vi "Obtain Priority Queue.vi"(8 "error in (no error)":errorcluster, 9 "Create If Not Found? (T)":bool=TRUE) -> (0 "error out":errorcluster, 1 "Created New?":bool, 3 "Priority Queue":T1)   [LabVIEW 2017, in "Communicable State Machine.lvlib"]
doc: "### Obtain Priority Queue.vi\n\n-- <b>Controls</b> --\n- <b>create if not found? (T)</b>:\n- <b>name</b>:\n\n-- <b>Indicators</b> --\n- <b>created new?</b>:\n- <b>Priority Queue</b>:"
uses:
  Communicable State Machine.lvlib
  Priority Queue.ctl
  Typedef/_Cross CSM State Data.ctl
  Typedef/_CSM_MSG_TYPE.ctl
  Typedef/_Cross CSM State Response.ctl
  Typedef/_CSM_Response Source Message.ctl
  def-Data(LowPRI-Q).ctl
panel:
  in  "Name":string
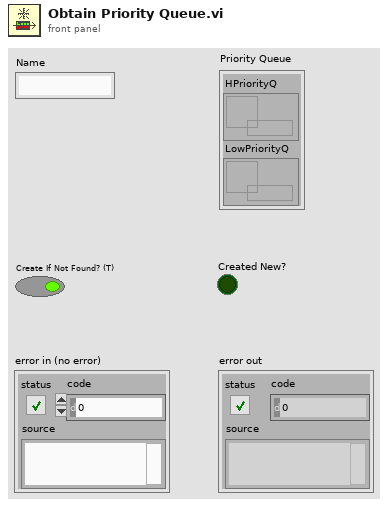
[diagram p1: front panel]
types:
  T1 = typedef "Communicable State Machine.lvlib/Priority Queue.ctl" = cluster{"HPriorityQ":refnum<queue>, "LowPriorityQ":refnum<queue>}
  T2 = typedef "Communicable State Machine.lvlib/def-Data(LowPRI-Q).ctl" = cluster{"Data":T3, "Notify?":bool}
  T3 = typedef "Communicable State Machine.lvlib/_Cross CSM State Data.ctl" = cluster{"Msg Type":T4, "state":string, "args":string, "source":string, "RespQ":refnum<queue>, "Response For Message":T5, "Target":string}
  T4 = typedef "Communicable State Machine.lvlib/_CSM_MSG_TYPE.ctl" = enum16{"Sync Message(-@)", "Async Message(->)", "Async without Response(->|)", "Async Response", "Broadcast(-><all>)", "Broadcast(-><status>)", "Broadcast(-><interrupt>)", "Append to JKISM States", "Append to JKISM States(High Priority)", "Broadcast(-><state>)"}
  T5 = typedef "Communicable State Machine.lvlib/_CSM_Response Source Message.ctl" = cluster{"‘State":string, "’Arguments":string, "’Error":errorcluster}
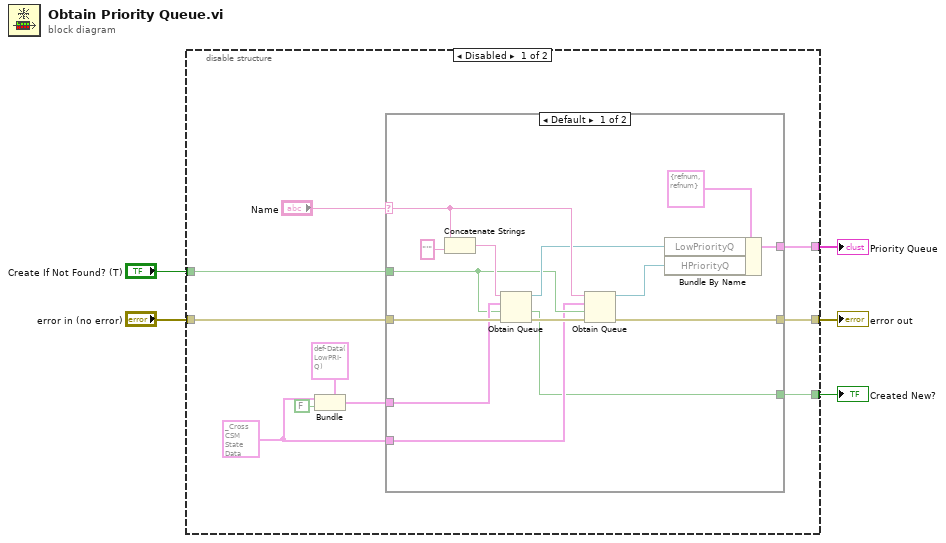
[diagram p0: block diagram]
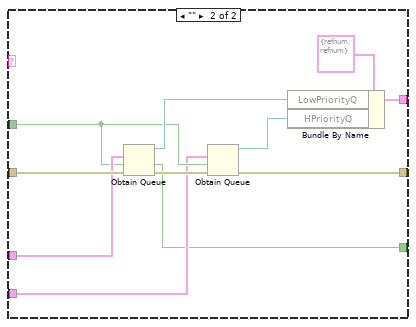
[diagram p2: hidden frame]
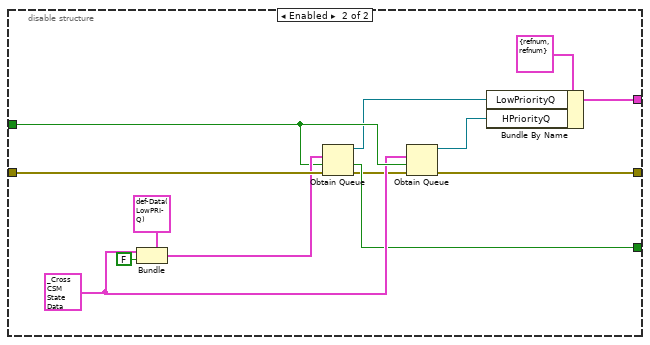
[diagram p3: hidden frame]
diagram:
  n1 = disable-structure shown="Disabled" {
    disable-tunnel: "error in (no error)" -> [w15 w53]
    disable-tunnel: [w14 w52] -> w4
    disable-tunnel: [w13 w51] -> w3
    disable-tunnel: "Create If Not Found? (T)" -> [w9 w47]
    disable-tunnel: [w7 w45] -> w1
    frame Disabled {
      w8 = T3 {"Msg Type"=enum."Sync Message(-@)", "state"="", "args"="", "source"="", "RespQ"=refnum, "Response For Message"={"‘State"="", "’Arguments"="", "’Error"={"status"=FALSE, "code"=0, "source"=""}}, "Target"=""} ("Cross JKI State Machine State")
      n2 = Bundle(cluster=T2 {"Data"={"Msg Type"=enum."Sync Message(-@)", "state"="", "args"="", "source"="", "RespQ"=refnum, "Response For Message"={"‘State"="", "’Arguments"="", "’Error"={"status"=FALSE, "code"=0, "source"=""}}, "Target"=""}, "Notify?"=FALSE}, "Data"=w8, "Notify?"=FALSE) -> (w11:T2)
      n3 = case shown="Default" "Name" {
        selector: "Name" -> [w27 _]
        tunnel: w15 -> [w29 w40]
        tunnel: [w25 w39] -> w14
        tunnel: [w24 w38] -> w13
        tunnel: w11 -> [w22 w36]
        tunnel: w9 -> [w20 w34]
        tunnel: w8 -> [w19 w32]
        tunnel: [w18 w31] -> w7
        frame Default {
          n4 = Concatenate Strings(w27, "'" ("string")) -> (w28:string)
          n5 = Obtain Queue(name (unnamed)=w28, element data type=w22, create if not found? (T)=w20, error in (no error)=w29) -> (queue out=w23:refnum<queue>, created new?=w18:bool, error out=w21:errorcluster)  [unwired: 1 in]
          n6 = Obtain Queue(name (unnamed)=w27, element data type=w19, create if not found? (T)=w20, error in (no error)=w21) -> (queue out=w17:refnum<queue>, error out=w24:errorcluster)  [unwired: 1 in, 1 out]
          n7 = Bundle By Name(cluster=T1 {"HPriorityQ"=refnum, "LowPriorityQ"=refnum} ("Priority Queue"), "LowPriorityQ"=w23, "HPriorityQ"=w17) -> (w25:T1)
        }
        frame "" {
          n8 = Obtain Queue(element data type=w36, create if not found? (T)=w34, error in (no error)=w40) -> (queue out=w37:refnum<queue>, created new?=w31:bool, error out=w35:errorcluster)  [unwired: 2 in]
          n9 = Obtain Queue(element data type=w32, create if not found? (T)=w34, error in (no error)=w35) -> (queue out=w30:refnum<queue>, error out=w38:errorcluster)  [unwired: 2 in, 1 out]
          n10 = Bundle By Name(cluster=T1 {"HPriorityQ"=refnum, "LowPriorityQ"=refnum} ("Priority Queue"), "LowPriorityQ"=w37, "HPriorityQ"=w30) -> (w39:T1)
        }
      }
    }
    frame Enabled {
      w46 = T3 {"Msg Type"=enum."Sync Message(-@)", "state"="", "args"="", "source"="", "RespQ"=refnum, "Response For Message"={"‘State"="", "’Arguments"="", "’Error"={"status"=FALSE, "code"=0, "source"=""}}, "Target"=""} ("Cross JKI State Machine State")
      n11 = Bundle(cluster=T2 {"Data"={"Msg Type"=enum."Sync Message(-@)", "state"="", "args"="", "source"="", "RespQ"=refnum, "Response For Message"={"‘State"="", "’Arguments"="", "’Error"={"status"=FALSE, "code"=0, "source"=""}}, "Target"=""}, "Notify?"=FALSE}, "Data"=w46, "Notify?"=FALSE) -> (w49:T2)
      n12 = Obtain Queue(element data type=w49, create if not found? (T)=w47, error in (no error)=w53) -> (queue out=w44:refnum<queue>, created new?=w45:bool, error out=w43:errorcluster)  [unwired: 2 in]
      n13 = Obtain Queue(element data type=w46, create if not found? (T)=w47, error in (no error)=w43) -> (queue out=w41:refnum<queue>, error out=w51:errorcluster)  [unwired: 2 in, 1 out]
      n14 = Bundle By Name(cluster=T1 {"HPriorityQ"=refnum, "LowPriorityQ"=refnum} ("Priority Queue"), "LowPriorityQ"=w44, "HPriorityQ"=w41) -> (w52:T1)
    }
  }
  "Priority Queue" <- w4
  "error out" <- w3
  "Created New?" <- w1
